vi "Read waveform type.vi"(8 "error in (no error)":errorcluster caption="에러 입력(에러 없음)", 11 "PWL 입력":refnum<class "PWL.lvclass">) -> (0 "error out":errorcluster caption="에러 출력", 2 "waveform type":T1, 3 "PWL 출력":refnum<class "PWL.lvclass">)   [LabVIEW 2020, in "PWL.lvclass"]
uses:
  PWL.lvclass
  Waveform Gen/Controls/waveform gen type.ctl
  PWL.lvclass/PWL.ctl
  Waveform Gen/Waveform Gen.lvclass
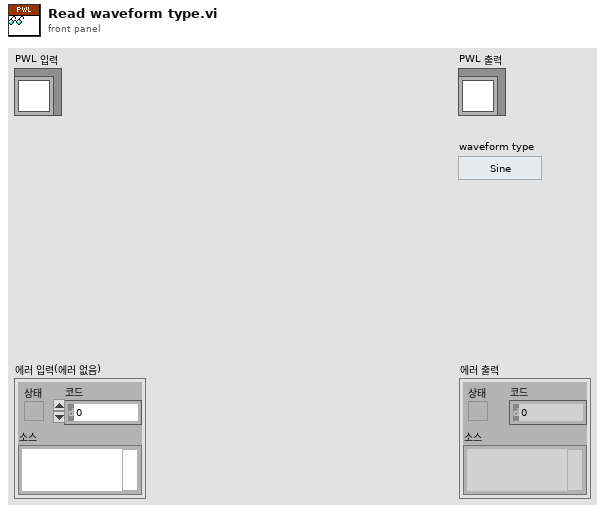
[diagram p1: front panel]
types:
  T1 = typedef "Waveform Gen.lvclass/waveform gen type.ctl" = enum16{"Sine", "Square", "Triangle", "Sawtooth", "Auto Track", "Auto Brake (Square)", "Auto Brake (Sine)", "PWL"}
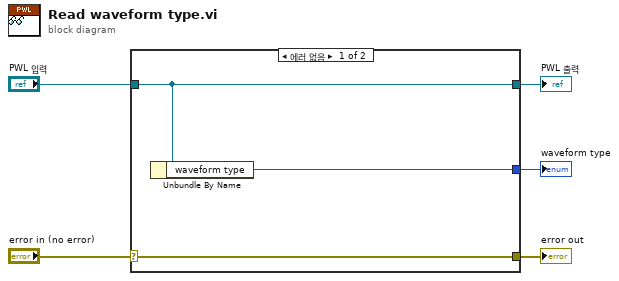
[diagram p0: block diagram]
diagram:
  n1 = case shown="에러 없음" "error in (no error)" {
    selector: "error in (no error)" -> [w8 w9]
    tunnel: [w8 w9] -> w4
    tunnel: [w7 w10] -> w2
    tunnel: "PWL 입력" -> [w7 w10]
    tunnel: [w6 _] -> w1
    frame No Error {
      n2 = Unbundle By Name(w7) -> ("waveform type"=w6:T1)
    }
    frame Error {
    }
  }
  "error out" <- w4
  "PWL 출력" <- w2
  "waveform type" <- w1
